vi "New_Counter.vi"   [LabVIEW 2015]
uses:
  <vilib>/DAQmx/create/channels.llb/DAQmx Create Channel (CI-Count Edges).vi
  <resource>/objmgr/daqmx.rc
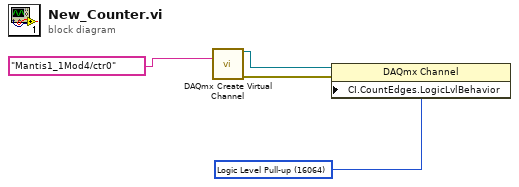
[diagram p0: block diagram]
diagram:
  w2 = 16064 items=["Logic Level Pull-up"=16064, "None"=10230] ("CI.CountEdges.LogicLvlBehavior")
  n1 = call-poly <vilib>:"DAQmx Create Virtual Channel.vi"("counter"=tag "Mantis1_1Mod4/ctr0") -> ("task out"=w3:refnum<k21>, "error out"=w1:errorcluster)  [unwired: 13 in]
  n2 = property class="DAQmx Channel"(reference=w3, error in=w1, "CI.CountEdges.LogicLvlBehavior"=w2) -> ()  [unwired: 2 out]
